vi "Process Buy.vi"(8 "error in (no error)":errorcluster, 11 "UI Actor in":refnum<class "UI Actor.lvclass">) -> (0 "error out":errorcluster, 3 "UI Actor out":refnum<class "UI Actor.lvclass">)   [LabVIEW 2020, in "UI Actor.lvlib" / "UI Actor.lvclass"]
uses:
  UI Actor.lvclass
  C:/Program Files/National Instruments/LabVIEW 2020/vi.lib/ActorFramework/Actor/Actor.lvclass
  <vilib>/ActorFramework/Actor/Actor.lvclass/Actor.ctl
  <vilib>/ActorFramework/Message Enqueuer/Message Enqueuer.lvclass/Message Enqueuer.ctl
  UI Actor.lvclass/UI Actor.ctl
  USD Actor Messages/Reset credit Msg/Reset credit Msg.lvclass/Reset credit Msg.ctl
  Msg Messages/Update MSG Msg/Update MSG Msg.lvclass/Update MSG Msg.ctl
  UI Actor Messages/Credit Update Msg/Credit Update Msg.lvclass/Credit Update Msg.ctl
  <vilib>/ActorFramework/Message Enqueuer/Init from Existing Queue.vi
  <vilib>/ActorFramework/Message Enqueuer/Enqueue.vi
  USD Actor Messages/Reset credit Msg/Reset credit Msg.lvclass
  C:/Program Files/National Instruments/LabVIEW 2020/vi.lib/ActorFramework/Message/Message.lvclass
  Msg Messages/Update MSG Msg/Update MSG Msg.lvclass
  UI Actor Messages/Credit Update Msg/Credit Update Msg.lvclass
  <vilib>/Utility/config.llb/Read Key (Double).vi
  <vilib>/ActorFramework/Message Priority Queue/Priority Enqueue.vi
  <vilib>/ActorFramework/Message Enqueuer/Message Enqueuer.lvclass
  <vilib>/Utility/config.llb/NI_LVConfig.lvlib
  <vilib>/ActorFramework/Actor/Actor.lvclass
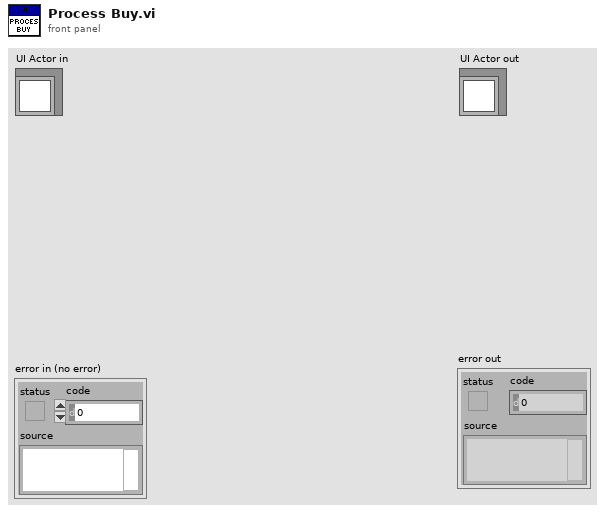
[diagram p1: front panel]
types:
  T1 = typedef "NI_LVConfig.lvlib/Config Data RefNum.ctl" = refnum<k1>
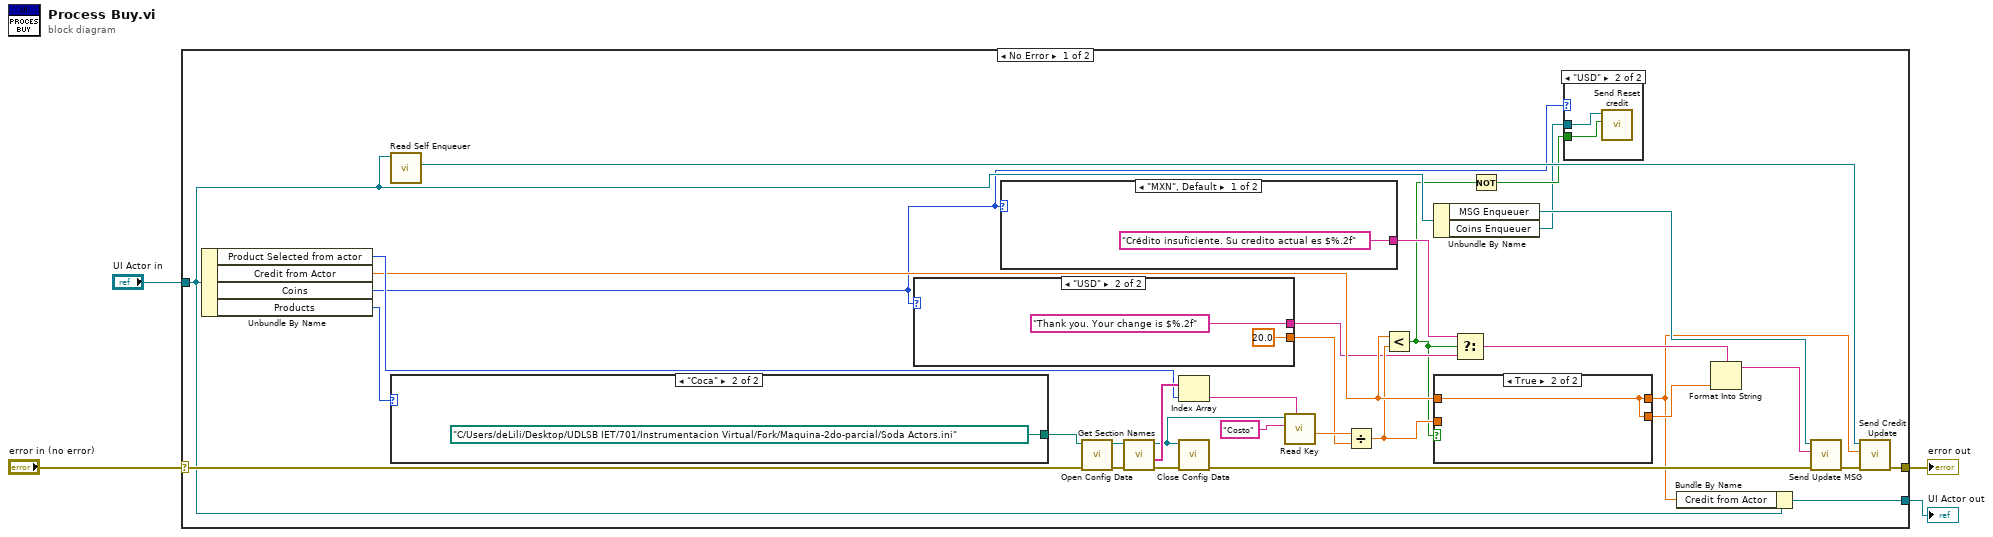
[diagram p0: block diagram]
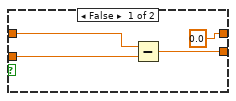
[diagram p3: hidden frame]
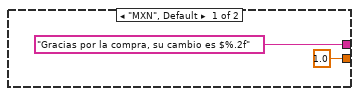
[diagram p4: hidden frame]
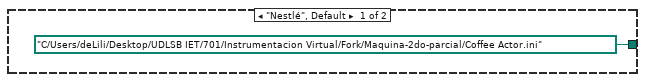
[diagram p5: hidden frame]
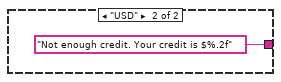
[diagram p6: hidden frame]
diagram:
  n1 = case shown="No Error" "error in (no error)" {
    selector: "error in (no error)" -> [w24 w53]
    tunnel: [w19 w53] -> w3
    tunnel: [w18 w52] -> w1
    tunnel: "UI Actor in" -> [w16 w52]
    frame No Error {
      n2 = Unbundle By Name(w16) -> ("Product Selected from actor"=w30:i32, "Credit from Actor"=w13:dbl, "Coins"=w8:enum16{"MXN", "USD"}, "Products"=w36:enum16{"Nestlé", "Coca"})
      n3 = call <vilib>:"Read Self Enqueuer.vi"("Actor"=w16) -> ("Self Enqueuer"=w17:refnum<class "Message Enqueuer.lvclass">)  [unwired: 10 in]
      n4 = case shown="\"Coca\"" w36 {
        tunnel: [path "C:/Users/deLili/Desktop/UDLSB IET/701/Instrumentacion Virtual/Fork/Maquina-2do-parcial/Coffee Actor.ini" ("configuration file path") path "C:/Users/deLili/Desktop/UDLSB IET/701/Instrumentacion Virtual/Fork/Maquina-2do-parcial/Soda Actors.ini" ("configuration file path")] -> w35
        frame "Nestlé", Default {
        }
        frame "Coca" {
        }
      }
      n5 = case shown="\"USD\"" w8 {
        tunnel: [1.0 ("y") 20.0 ("y")] -> w25
        tunnel: ["Gracias por la compra, su cambio es $%.2f" ("format string") "Thank you. Your change is $%.2f" ("format string")] -> w10
        frame "MXN", Default {
        }
        frame "USD" {
        }
      }
      n6 = case shown="\"MXN\", Default" w8 {
        tunnel: ["Crédito insuficiente. Su credito actual es $%.2f" ("format string") "Not enough credit. Your credit is $%.2f" ("format string")] -> w9
        frame "MXN", Default {
        }
        frame "USD" {
        }
      }
      n7 = call <vilib>:"Open Config Data.vi"("error in (no error)"=w24, "configuration file path"=w35) -> ("error out"=w34:errorcluster, "refnum"=w33:T1)  [unwired: 7 in, 1 out]
      n8 = call <vilib>:"Get Section Names.vi"("error in (no error)"=w34, "refnum"=w33) -> ("error out"=w32:errorcluster, "section names"=w31:string[], "refnum out"=w29:T1)  [unwired: 7 in]
      n9 = Index Array(array=w31, index=w30) -> (element=w28:string)
      n10 = call <vilib>:"Close Config Data.vi"("error in (no error)"=w32, "refnum"=w29) -> ("error out"=w21:errorcluster)  [unwired: 8 in, 1 out]
      n11 = call-poly <vilib>:"Read Key.vi"("section"=w28, "key"="Costo", "refnum"=w29) -> ("value"=w26:dbl)  [unwired: 5 in, 3 out]
      n12 = Divide(x=w26, y=w25) -> (x/y=w12:dbl)
      n13 = Less?(x=w13, y=w12) -> (x < y?=w7:bool)
      n14 = Unbundle By Name(w16) -> ("MSG Enqueuer"=w15:refnum<class "Message Enqueuer.lvclass">, "Coins Enqueuer"=w5:refnum<class "Message Enqueuer.lvclass">)
      n15 = case shown="True" w7 {
        tunnel: [w42 w43] -> w23
        tunnel: w13 -> [w41 w43]
        tunnel: w12 -> [w40 _]
        tunnel: [0.0 ("Credit") w43] -> w11
        frame False {
          n16 = Subtract(x=w41, y=w40) -> (x-y=w42:dbl)
        }
        frame True {
        }
      }
      n17 = Select(t=w9, s=w7, f=w10) -> (s? t:f=w14:string)
      n18 = Not(x=w7) -> (.not. x?=w6:bool)
      n19 = case shown="\"USD\"" w8 {
        tunnel: w6 -> [_ w38]
        tunnel: w5 -> [_ w37]
        frame "MXN", Default {
        }
        frame "USD" {
          n20 = call "Send Reset credit.vi"("Compra realizada?"=w38, "Message Enqueuer"=w37) -> ()  [unwired: 8 in, 2 out]
        }
      }
      n21 = Bundle By Name(cluster=w16, "Credit from Actor"=w11) -> (w18:refnum<class "UI Actor.lvclass">)
      n22 = Format Into String(format string=w14, w23) -> (resulting string=w22:string)  [unwired: 2 in, 1 out]
      n23 = call "Send Update MSG.vi"("error in (no error)"=w21, "Update MSG"=w22, "Message Enqueuer"=w15) -> ("error out"=w20:errorcluster)  [unwired: 7 in, 1 out]
      n24 = call "Send Credit Update.vi"("error in (no error)"=w20, "Credit"=w11, "Message Enqueuer"=w17) -> ("error out"=w19:errorcluster)  [unwired: 7 in, 1 out]
    }
    frame Error {
    }
  }
  "error out" <- w3
  "UI Actor out" <- w1
